vi "RDV-autoscale.vi"(8 "error in (no error)":errorcluster, 10 "Autoscale":bool, 11 "RDV-Reflection_Data_viewer in":refnum<class "RDV-Reflection_Data_viewer.lvclass">) -> (0 "error out":errorcluster, 3 "RDV-Reflection_Data_viewer out":refnum<class "RDV-Reflection_Data_viewer.lvclass">)   [LabVIEW 2020, in "RDV-Reflection_Data_viewer.lvclass"]
uses:
  RDV-Reflection_Data_viewer.lvclass
  RDV-Reflection_Data_viewer.lvclass/RDV-Reflection_Data_viewer.ctl
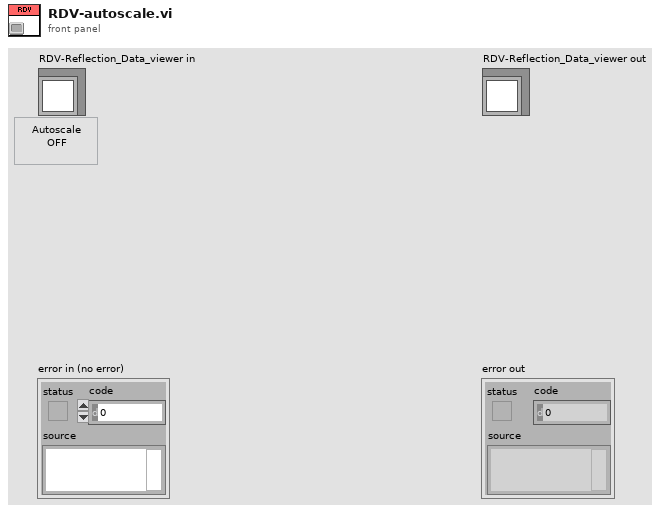
[diagram p1: front panel]
types:
  T1 = typedef "RDV-Reflection_Data_viewer.lvclass/RDV-XY_GRAPH_REFS.ctl" = cluster{"Reflection Real":refnum<vi>, "Reflection Imag":refnum<vi>, "Permittivity Real":refnum<vi>, "Permittivity Imag":refnum<vi>}
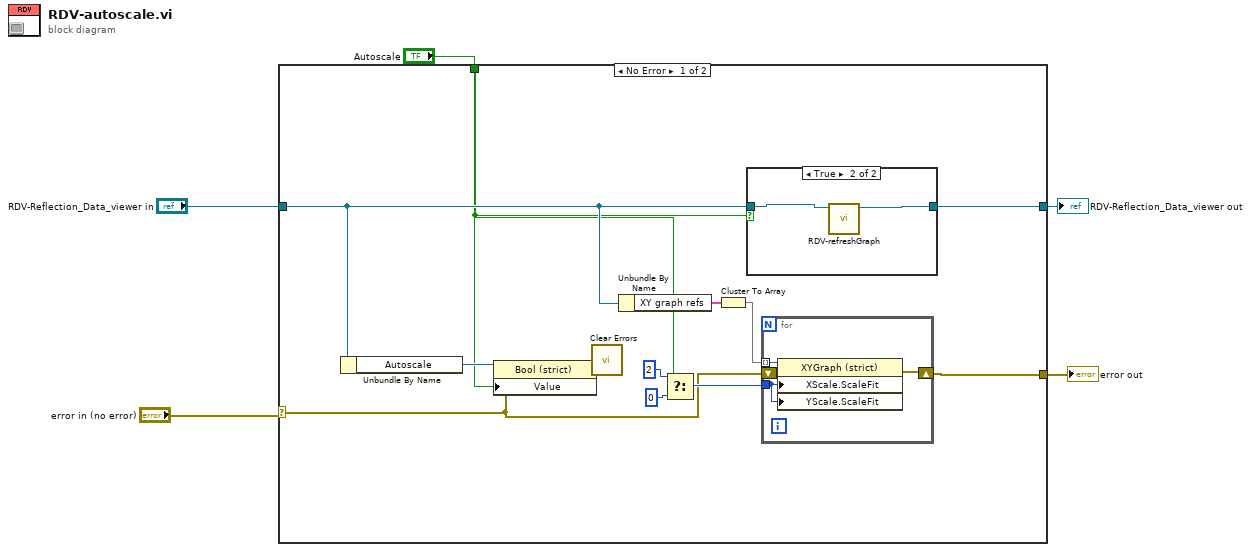
[diagram p0: block diagram]
diagram:
  n1 = case shown="No Error" "error in (no error)" {
    selector: "error in (no error)" -> [w10 w26]
    tunnel: [w11 w26] -> w4
    tunnel: [w6 w25] -> w2
    tunnel: "RDV-Reflection_Data_viewer in" -> [w8 w25]
    tunnel: "Autoscale" -> [w7 _]
    frame No Error {
      n2 = Unbundle By Name(w8) -> ("Autoscale"=w17:refnum<vi>)
      n3 = property class="Bool (strict)"(reference=w17, error in=w10, "Value"=w7) -> (error out=w9:errorcluster)  [unwired: 1 out]
      n4 = call <vilib>:"Clear Errors.vi"("error in (no error)"=w9) -> ()  [unwired: 5 in, 2 out]
      n5 = Unbundle By Name(w8) -> ("XY graph refs"=w16:T1)
      n6 = Select(t=u8 2 ("X Scale.Scale Fit"), s=w7, f=u8 0 ("X Scale.Scale Fit")) -> (s? t:f=w12:u8)
      n7 = Cluster To Array(cluster=w16) -> (array=w15:refnum<vi>[])
      n8 = case shown="True" w7 {
        tunnel: w8 -> [w18 w20]
        tunnel: [w18 w19] -> w6
        frame False {
        }
        frame True {
          n9 = call "RDV-refreshGraph.vi"("RDV-Reflection_Data_viewer in"=w20) -> ("RDV-Reflection_Data_viewer out"=w19:refnum<class "RDV-Reflection_Data_viewer.lvclass">)  [unwired: 9 in, 1 out]
        }
      }
      n10 = for {
        tunnel: w15 -> [w24] mode=indexing
        tunnel: w12 -> [w21]
        shift-right: [w22] -> w11
        shift-left: w10 -> [w23]
        n11 = property class="XYGraph (strict)"(reference=w24, error in=w23, "XScale.ScaleFit"=w21, "YScale.ScaleFit"=w21) -> (error out=w22:errorcluster)  [unwired: 1 out]
      }
    }
    frame Error {
    }
  }
  "error out" <- w4
  "RDV-Reflection_Data_viewer out" <- w2
